vi "Get Type.vi"(8 "error in (no error)":errorcluster, 11 "Simple Circuit in":refnum<class "Simple Circuit.lvclass">) -> (0 "error out":errorcluster, 2 "Item Type":T1, 3 "Simple Circuit out":refnum<class "Simple Circuit.lvclass">)   [LabVIEW 2020, in "Simple Circuit.lvclass"]
uses:
  Simple Circuit.lvclass
  Item/Item Type.ctl
  Item/Item.lvclass
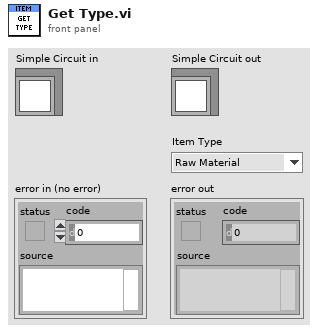
[diagram p1: front panel]
types:
  T1 = typedef "Item.lvclass/Item Type.ctl" = enum16{"Raw Material", "Component", "Module", "Product"}
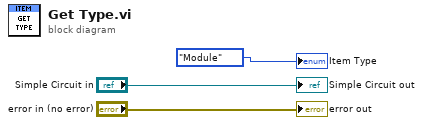
[diagram p0: block diagram]
diagram:
  "error out" <- "error in (no error)"
  "Simple Circuit out" <- "Simple Circuit in"
  "Item Type" <- Item_Type."Module" ("Item Type")
